vi "Write Output Channels.vi"(8 "error in (no error)":errorcluster, 9 "Status":dbl, 10 "Outputs":T1, 11 "Device Outputs FIFO":refnum<k33>) -> (0 "error out":errorcluster, 2 "Updated Outputs":T1)   [LabVIEW 2017, in "SLSC Switch Engine.lvlib"]
uses:
  SLSC Switch Engine.lvlib
  Outputs With Indices.ctl
  Shared/FIFO Indices.ctl
  Shared/SLSC Switch Shared.lvlib
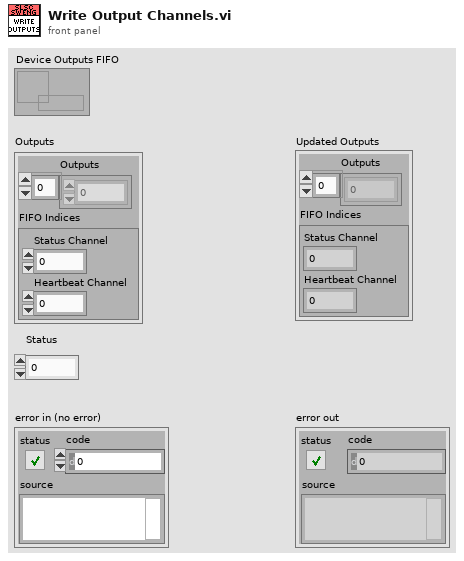
[diagram p1: front panel]
types:
  T1 = typedef "SLSC Switch Engine.lvlib/Outputs With Indices.ctl" = cluster{"Outputs":dbl[], "FIFO Indices":T2}
  T2 = typedef "SLSC Switch Shared.lvlib/FIFO Indices.ctl" = cluster{"Status Channel":i32, "Heartbeat Channel":i32}
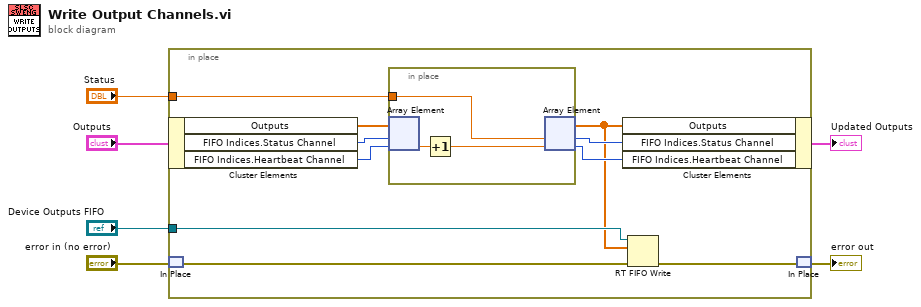
[diagram p0: block diagram]
diagram:
  n1 = in-place {
    in-place-border: "Status" -> [w11]
    in-place-border: "Device Outputs FIFO" -> [w10]
    n2 = in-place-cluster #1("Outputs") -> ("Outputs"=w16:dbl[], "FIFO Indices.Status Channel"=w15:i32, "FIFO Indices.Heartbeat Channel"=w14:i32)
    n3 = in-place-match #2("error in (no error)") -> (w8:errorcluster)
    n4 = in-place {
      in-place-border: w11 -> [w17]
      n5 = in-place-array #3(w16, w15, w14) -> (w19:dbl)  [unwired: 1 out]
      n6 = Increment(x=w19) -> (x+1=w18:dbl)
      n7 = in-place-array #3(w17, w18) -> (w9:dbl[], w13:i32, w12:i32)
    }
    n8 = in-place-cluster #1("Outputs"=w9, "FIFO Indices.Status Channel"=w13, "FIFO Indices.Heartbeat Channel"=w12) -> (→"Updated Outputs":T1)
    n9 = RT FIFO Write(0:w10, 1:w9, 3:w8) -> (11:w7:errorcluster)  [unwired: 1 in, 4 out]
    n10 = in-place-match #2(w7) -> (→"error out":errorcluster)
  }
